vi "Buffer Overflow Solution.vi"() -> ()   [LabVIEW 2010]
uses:
  <vilib>/express/express analysis/Spectral/XNode/ExpressSpectralMeasurementsBlockNode.xnode
  Instance           1 32Saved   Buffer Overflow Solution .vi
  Instance           5 32Saved   Buffer Overflow Solution .vi
  Instance           4 32Saved   Buffer Overflow Solution .vi
  <vilib>/express/express analysis/Spectral/Block/exnSpectralBlock spectral measurements power poly.vi
  <vilib>/express/express analysis/Spectral/Block/exnSpectralBlock spectral measurements power DDT.vi
  Program Files/National Instruments/LabVIEW 2010/resource/objmgr/daqmx.rc
panel:
  out "주파수":dbl
  out "큐 크기":i32
  in  "모형 컨트롤":dynamicdata(graph)
  out "DAQ 버퍼 크기":u32
  out "파워 스펙트럼":dynamicdata(graph)
  in  "정지":bool
  out "시간 데이터":dynamicdata(graph)
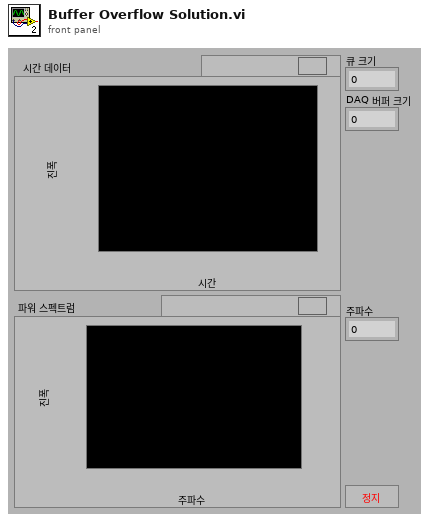
[diagram p1: front panel]
types:
  T1 = cluster{"averaging mode":u16, "weighting mode":u16, "number of averages":u32}
  T2 = cluster{"dB On (F)":bool, "unwrap phase (F)":bool, "convert to degree (F)":bool}
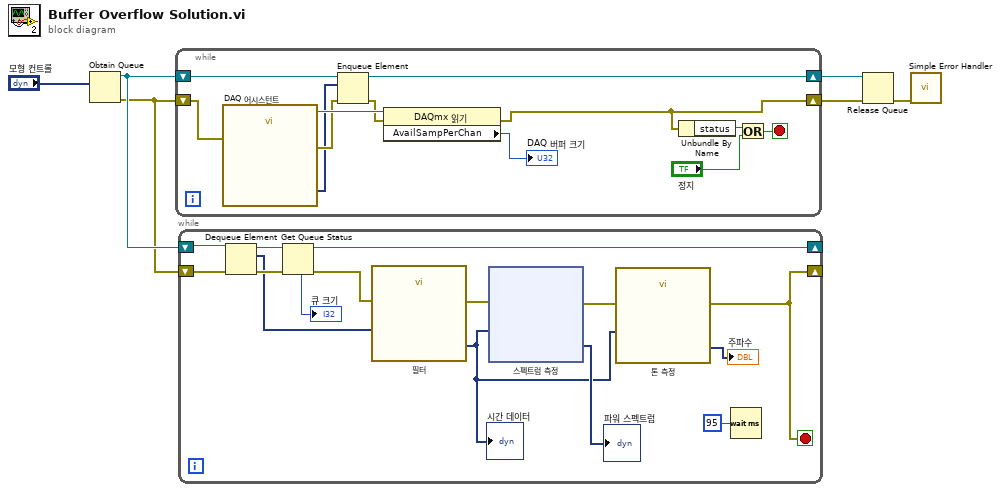
[diagram p0: block diagram]
diagram:
  n1 = Obtain Queue(element data type="모형 컨트롤") -> (queue out=w6:refnum<queue>, error out=w4:errorcluster)  [unwired: 4 in, 1 out]
  n2 = while {
    shift-right: [w7] -> w2
    shift-left: w4 -> [w13]
    shift-right: [w8] -> w3
    shift-left: w6 -> [w12]
    stop <- w15 stop-if-true
    n3 = call "DAQ 어시스턴트"("error in"=w13) -> ("task out"=w18:refnum<k21>, "data"=w9:dynamicdata, "error out"=w11:errorcluster)  [unwired: 15 in, 1 out]
    n4 = Enqueue Element(queue=w12, element=w9, error in (no error)=w11) -> (queue out=w8:refnum<queue>, error out=w10:errorcluster)  [unwired: 1 in, 1 out]
    n5 = property class="DAQmx 읽기"(reference=w18, error in=w10) -> (error out=w7:errorcluster, "AvailSampPerChan"=→"DAQ 버퍼 크기":u32)  [unwired: 1 out]
    n6 = Unbundle By Name(w7) -> ("status"=w17:bool)
    n7 = Or(x=w17, y="정지") -> (x .or. y?=w15:bool)
  }
  n8 = while {
    shift-right: [w28] -> _
    shift-left: w6 -> [w33]
    shift-right: [w26] -> _
    shift-left: w4 -> [w30]
    stop <- w26 stop-if-true
    n9 = Dequeue Element(queue=w33, error in (no error)=w30) -> (queue out=w29:refnum<queue>, element=w22:dynamicdata, error out=w31:errorcluster)  [unwired: 1 in, 1 out]
    n10 = Get Queue Status(queue=w29, error in (no error)=w31) -> (queue out=w28:refnum<queue>, error out=w19:errorcluster, # elements in queue=→"큐 크기":i32)  [unwired: 1 in, 5 out]
    n11 = call "필터"("error in (no error)"=w19, "Signal"=w22) -> ("error out"=w20:errorcluster, "Filtered Signal"=w21:dynamicdata)  [unwired: 8 in]
    "시간 데이터" <- w21
    n12 = xnode "스펙트럼 측정"("신호"=w21, "에러 입력(에러 없음)"=w20) -> ("파워 스펙트럼"=→"파워 스펙트럼":dynamicdata, "에러 출력"=w32:errorcluster)
    n13 = call "톤 측정"("error in (no error)"=w32, "Signals"=w21) -> ("error out"=w26:errorcluster, "Frequency"=→"주파수":dynamicdata)  [unwired: 8 in]
    n14 = Wait (ms)(milliseconds to wait=u32 95) -> ()  [unwired: 1 out]
  }
  n15 = Release Queue(queue=w3, error in (no error)=w2) -> (error out=w1:errorcluster)  [unwired: 1 in, 2 out]
  n16 = call <vilib>:"Simple Error Handler.vi"("error in (no error)"=w1) -> ()  [unwired: 4 in, 5 out]
